vi "Main.vi"(8 "error in (no error)":errorcluster, 11 "ServiceManagerLoader in":refnum<class "ServiceManagerLoader.lvclass">) -> (0 "error out":errorcluster, 3 "ServiceManagerLoader out":refnum<class "ServiceManagerLoader.lvclass">)   [LabVIEW 2012, in "ServiceManagerLoader.lvclass"]
doc: "Main VI of the component."
uses:
  ServiceManagerLoader.lvclass
  Murmex/LabVIEW/Murmex/Murmex/Murmex.lvclass
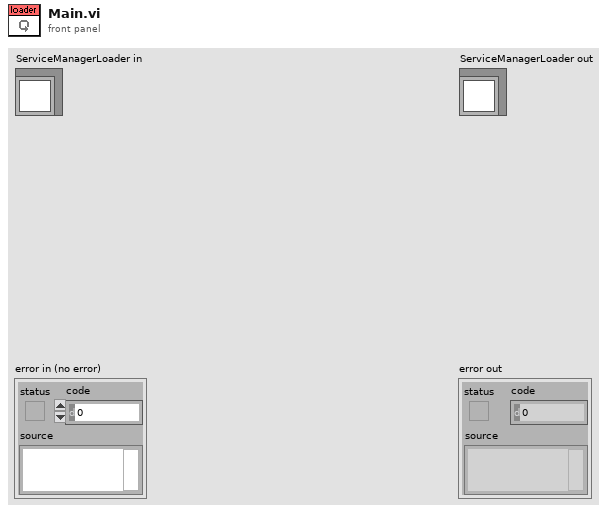
[diagram p1: front panel]
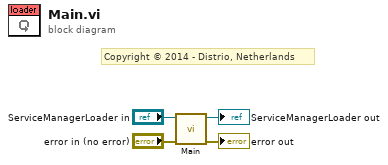
[diagram p0: block diagram]
diagram:
  # "Copyright © 2014 - Distrio, Netherlands"
  n1 = call-parent "Main.vi"("error in (no error)"="error in (no error)", "Murmex in"="ServiceManagerLoader in") -> ("error out"=→"error out":errorcluster, "Murmex out"=→"ServiceManagerLoader out":refnum<class "ServiceManagerLoader.lvclass">)  [unwired: 8 in]
